vi "Test RT-TDMS-Logging API.vi"() -> ()   [LabVIEW 2021]
doc: "RT-TDMS-Logging API Tester."
uses:
  <vilib>/Utility/error.llb/DialogType.ctl
  RT-TDMS-Logging.lvlib
panel:
  in  "DO Data 2":variant
  in  "DO Data":bool
  in  "Start Logging 2":variant
  in  "Start Logging":bool
  in  "AI Data's 2":variant
  in  "AI Data's":bool
  in  "Data Logging Duration(Sec)":dbl
  in  "Data Logging Duration":bool
  out "last error":errorcluster
  in  "Show Diagram on Init":bool
  in  "Show Block Diagram":bool
  in  "Stop Module":bool
  in  "Start Module":bool
  in  "Hide Module Panel":bool
  in  "Show Module Panel":bool
  out "Status":string
  out "Module Running?":bool
  # "This VI tests the API for the Module."
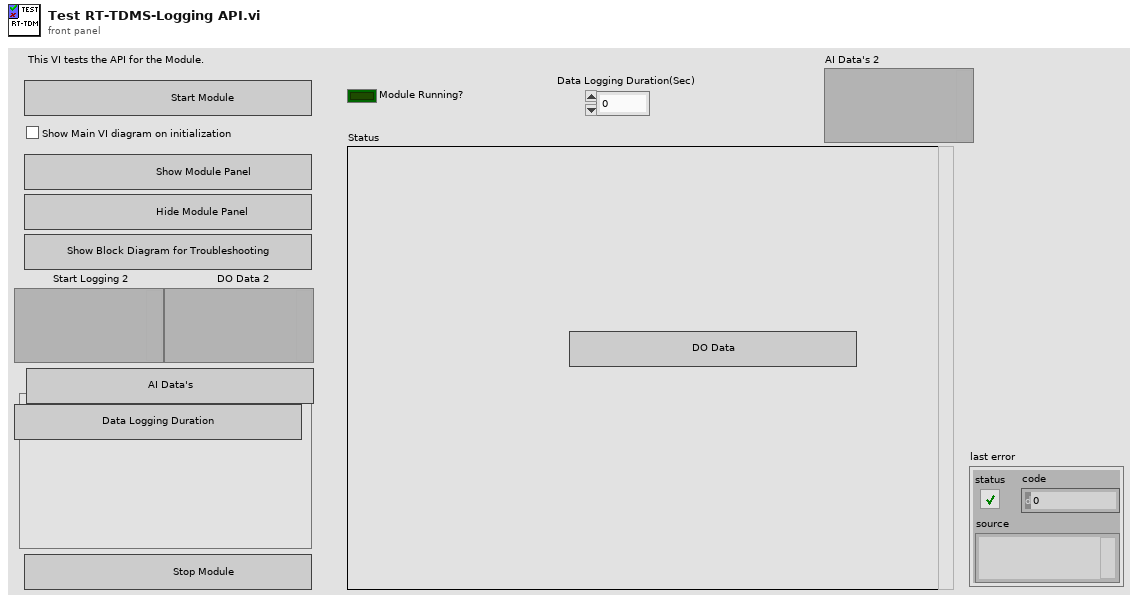
[diagram p1: front panel]
types:
  T1 = typedef "RT-TDMS-Logging.lvlib/Broadcast Events--cluster.ctl" = cluster{"Module Did Init":refnum<user-event>, "Status Updated":refnum<user-event>, "Error Reported":refnum<user-event>, "Module Did Stop":refnum<user-event>, "Update Module Execution Status":refnum<user-event>}
  T2 = typedef "DialogType.ctl" = u16
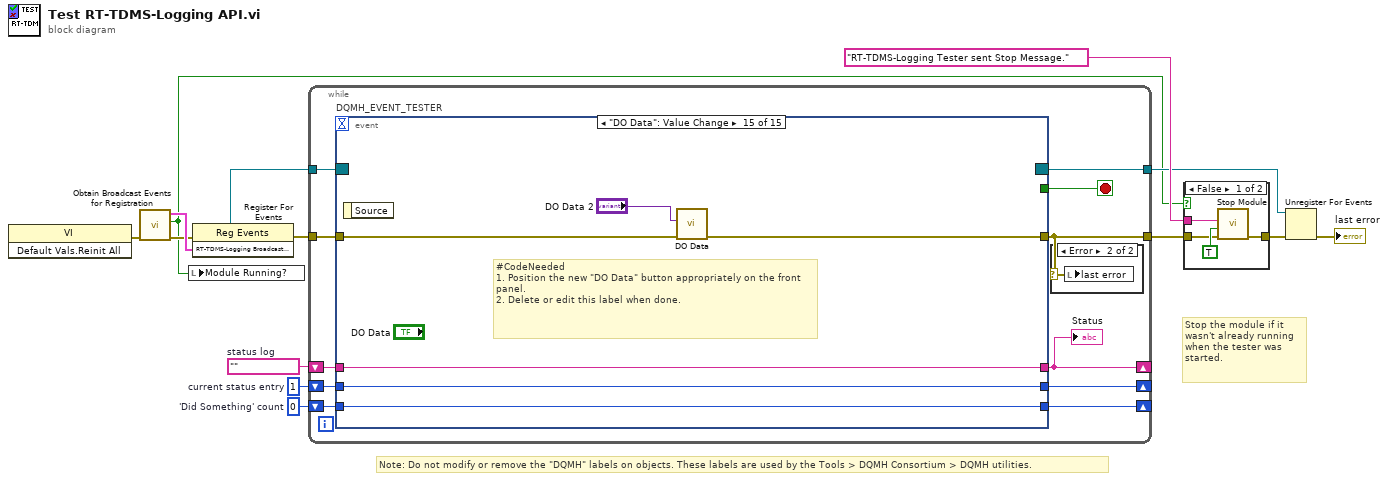
[diagram p0: block diagram]
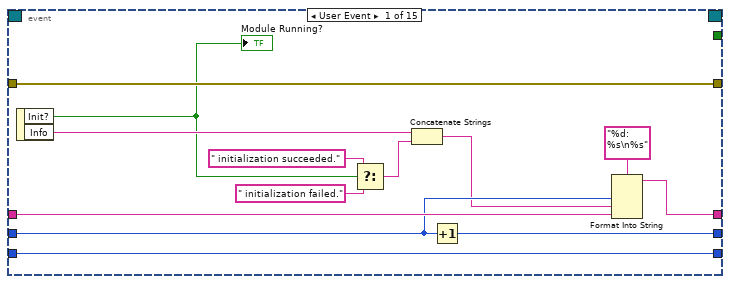
[diagram p4: hidden frame]
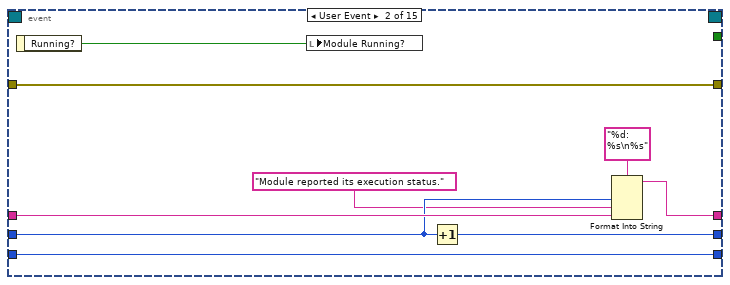
[diagram p5: hidden frame]
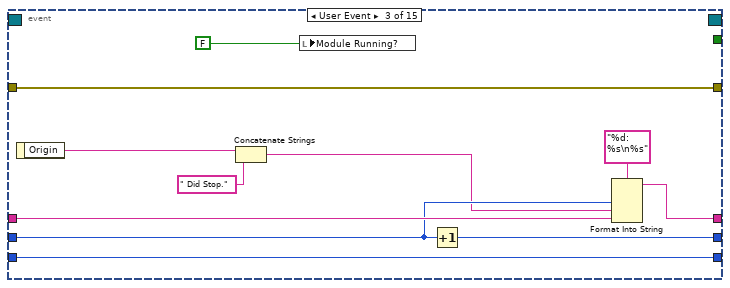
[diagram p6: hidden frame]
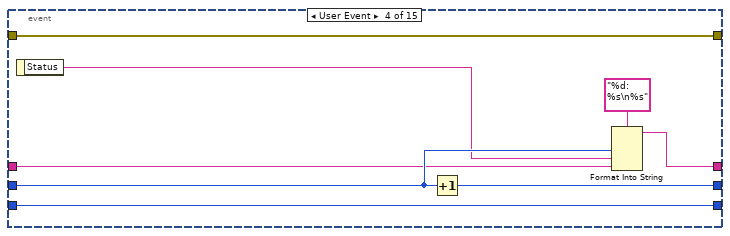
[diagram p7: hidden frame]
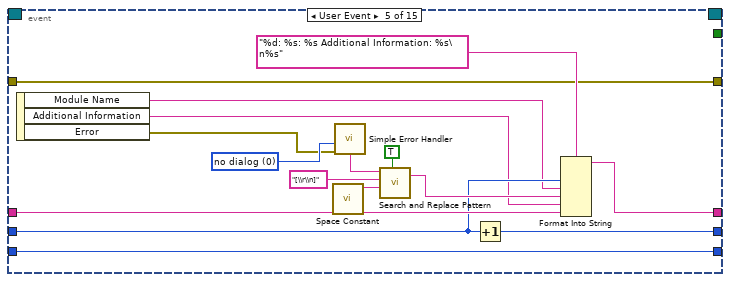
[diagram p8: hidden frame]
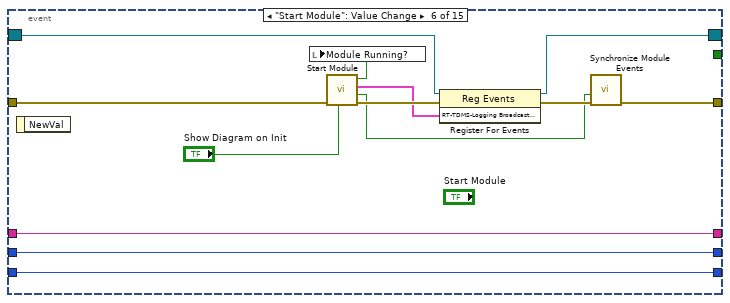
[diagram p9: hidden frame]
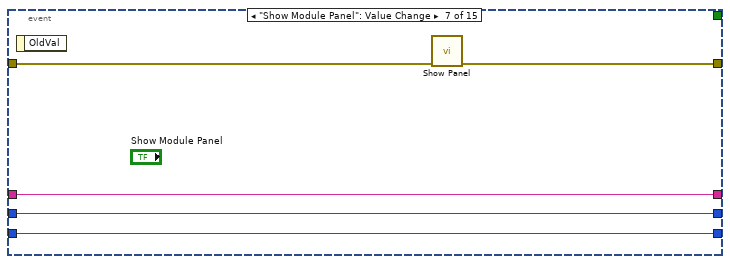
[diagram p10: hidden frame]
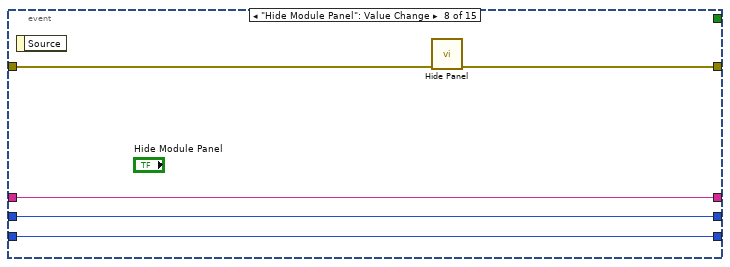
[diagram p11: hidden frame]
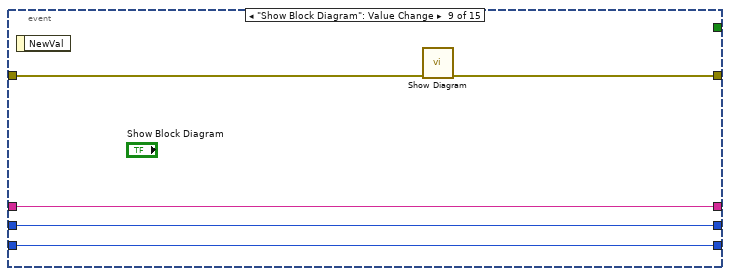
[diagram p12: hidden frame]
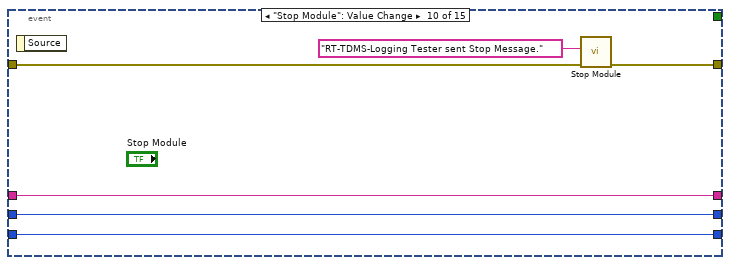
[diagram p13: hidden frame]
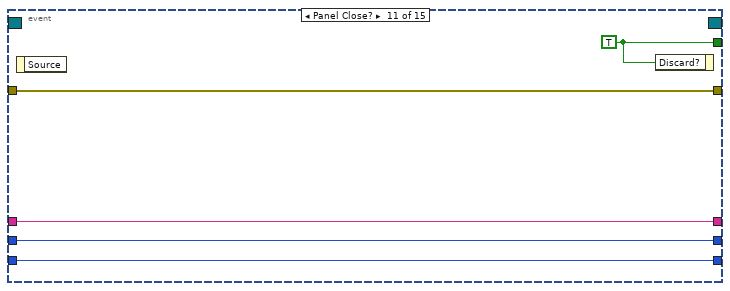
[diagram p14: hidden frame]
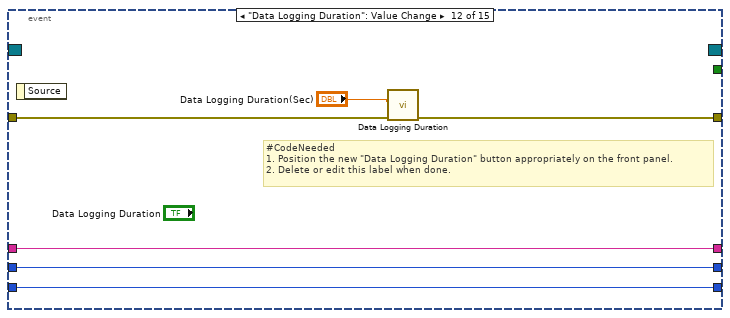
[diagram p15: hidden frame]
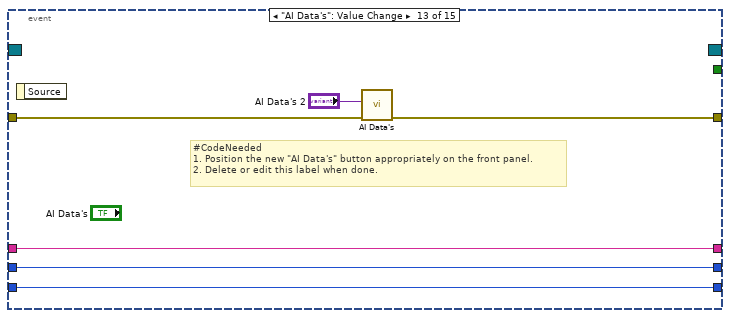
[diagram p16: hidden frame]
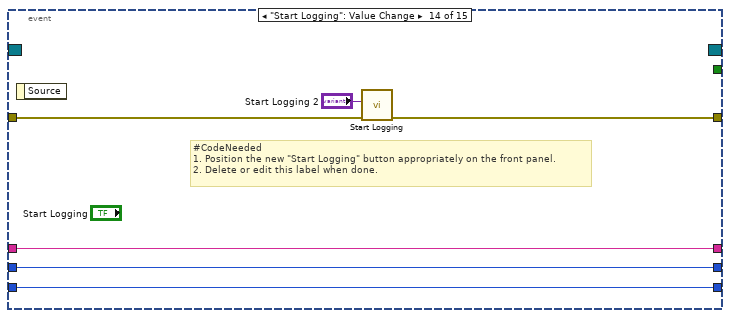
[diagram p17: hidden frame]
diagram:
  w10 = 0  # 'Did Something' count
  w11 = 1  # current status entry
  w12 = ""  # status log
  # "Stop the module if it wasn't already running when the tester was started."
  # "Note: Do not modify or remove the \"DQMH\" labels on objects. These labels are used by the Tools > DQMH Consortium > DQMH utilities."
  n1 = invoke class="VI" method="Default Vals.Reinit All"() -> (error out=w5:errorcluster)  [unwired: 3 in, 2 out]
  n2 = call "Obtain Broadcast Events for Registration.vi"("error in"=w5) -> ("error out"=w4:errorcluster, "Already running?"=w3:bool, "RT-TDMS-Logging Broadcast Events"=w8:T1)  [unwired: 8 in]
  n3 = local write "Module Running?"(w3) -> ()
  n4 = register-events(error in=w4, w8) -> (reference out=w7:refnum<event-registration>, error out=w9:errorcluster)  [unwired: 1 in]
  n5 = while {
    tunnel: w7 -> [w25]
    tunnel: [w15] -> w2
    shift-right: [w21] -> _
    shift-left: w12 -> [w23]
    shift-right: [w22] -> _
    shift-left: w11 -> [w24]
    shift-right: [w19] -> _
    shift-left: w10 -> [w20]
    tunnel: w9 -> [w18]
    tunnel: [w17] -> w6
    stop <- w16 stop-if-true
    n6 = event "DQMH_EVENT_TESTER" shown="[14] \"DO Data\": Value Change" {
      selector: w25 -> [_ _ _ _ _ w89 _ _ _ _ _ _ _ _ _]
      dyn-events: [_ _ _ _ _ w88 _ _ _ _ _ _ _ _ _] -> w17
      timeout: _ -> [_ _ _ _ _ _ _ _ _ _ _ _ _ _ _]
      tunnel: [_ _ _ _ _ _ _ _ _ _ w122 _ _ _ _] -> w16
      tunnel: [w39 w41 w49 w60 w71 w87 w101 w106 w107 w114 w118 w124 w130 w136 w142] -> w15
      tunnel: w24 -> [w36 w46 w57 w64 w74 w93 w99 w104 w109 w116 w120 w126 w132 w138 w144]
      tunnel: w23 -> [w37 w47 w58 w63 w75 w94 w100 w105 w110 w117 w121 w127 w133 w139 w145]
      tunnel: [w34 w44 w55 w65 w73 w94 w100 w105 w110 w117 w121 w127 w133 w139 w145] -> w21
      tunnel: [w35 w45 w56 w67 w72 w93 w99 w104 w109 w116 w120 w126 w132 w138 w144] -> w22
      tunnel: w20 -> [w31 w42 w51 w61 w83 w92 w98 w103 w108 w115 w119 w125 w131 w137 w143]
      tunnel: [w31 w42 w51 w61 w83 w92 w98 w103 w108 w115 w119 w125 w131 w137 w143] -> w19
      tunnel: w18 -> [w39 w41 w49 w60 w71 w86 w97 w102 w111 w112 w118 w128 w134 w140 w146]
      event User Event {
        n7 = event-data() -> ("Init?"=w30:bool, "Info"=w33:string)  [unwired: 1 in]
        "Module Running?" <- w30
        n8 = Select(t=" initialization succeeded.", s=w30, f=" initialization failed.") -> (s? t:f=w27:string)
        n9 = Concatenate Strings(w33, w27) -> (w32:string)
        n10 = Increment(x=w36) -> (x+1=w35:i32)
        n11 = Format Into String(format string="%d: %s\n%s", w36, w32, w37) -> (resulting string=w34:string)  [unwired: 2 in, 1 out]
      }
      event User Event {
        n12 = event-data() -> ("Running?"=w40:bool)  [unwired: 1 in]
        n13 = local write "Module Running?"(w40) -> ()
        n14 = Increment(x=w46) -> (x+1=w45:i32)
        n15 = Format Into String(format string="%d: %s\n%s", w46, "Module reported its execution status.", w47) -> (resulting string=w44:string)  [unwired: 2 in, 1 out]
      }
      event User Event {
        n16 = event-data() -> ("Origin"=w54:string)  [unwired: 1 in]
        n17 = Concatenate Strings(w54, " Did Stop.") -> (w53:string)
        n18 = local write "Module Running?"(FALSE ("Module Did Init?")) -> ()
        n19 = Increment(x=w57) -> (x+1=w56:i32)
        n20 = Format Into String(format string="%d: %s\n%s", w57, w53, w58) -> (resulting string=w55:string)  [unwired: 2 in, 1 out]
      }
      event User Event {
        n21 = event-data() -> ("Status"=w62:string)  [unwired: 1 in]
        n22 = Increment(x=w64) -> (x+1=w67:i32)
        n23 = Format Into String(format string="%d: %s\n%s", w64, w62, w63) -> (resulting string=w65:string)  [unwired: 2 in, 1 out]
      }
      event User Event {
        w76 = T2 0 items=["no dialog", "OK message", "continue or stop message", "OK message + warnings", "continue/stop + warnings"] ("type of dialog (OK msg:1)")
        n24 = event-data() -> ("Module Name"=w70:string, "Additional Information"=w69:string, "Error"=w68:errorcluster)  [unwired: 1 in]
        n25 = call <vilib>:"Space Constant.vi"() -> ("String"=w80:string)
        n26 = call <vilib>:"Simple Error Handler.vi"("type of dialog (OK msg:1)"=w76, "error in (no error)"=w68) -> ("message"=w77:string)  [unwired: 3 in, 4 out]
        n27 = call <vilib>:"Search and Replace Pattern.vi"("string"=w77, "regular expression (\"\")"="[\\r\\n]" ("regular expression (\"\")"), "replace string (\"\")"=w80, "replace all? (F)"=TRUE ("replace all CR/LF with spaces")) -> ("result string"=w78:string)  [unwired: 1 in, 1 out]
        n28 = Increment(x=w74) -> (x+1=w72:i32)
        n29 = Format Into String(format string="%d: %s: %s Additional Information: %s\n%s", w74, w70, w78, w69, w75) -> (resulting string=w73:string)  [unwired: 2 in, 1 out]
      }
      event "Start Module": Value Change {
        n30 = event-data() -> ()  [unwired: 1 in, 1 out]
        n31 = call "Start Module.vi"("Show Main VI Diagram on Init (F)"="Show Diagram on Init", "error in"=w86) -> ("error out"=w95:errorcluster, "Wait for Event Sync?"=w91:bool, "RT-TDMS-Logging Broadcast Events"=w90:T1, "Module Was Already Running?"=w85:bool)  [unwired: 6 in]
        n32 = local write "Module Running?"(w85) -> ()
        n33 = register-events(reference=w89, error in=w95, w90) -> (reference out=w88:refnum<event-registration>, error out=w96:errorcluster)
        n34 = call "Synchronize Module Events.vi"("error in"=w96, "Wait for Event Sync?"=w91) -> ("error out"=w87:errorcluster)  [unwired: 9 in]
      }
      event "Show Module Panel": Value Change {
        n35 = event-data() -> ()  [unwired: 1 in, 1 out]
        n36 = call "Show Panel.vi"("error in"=w97) -> ("error out"=w101:errorcluster)  [unwired: 10 in]
      }
      event "Hide Module Panel": Value Change {
        n37 = event-data() -> ()  [unwired: 1 in, 1 out]
        n38 = call "Hide Panel.vi"("error in"=w102) -> ("error out"=w106:errorcluster)  [unwired: 10 in]
      }
      event "Show Block Diagram": Value Change {
        n39 = event-data() -> ()  [unwired: 1 in, 1 out]
        n40 = call "Show Diagram.vi"("error in"=w111) -> ("error out"=w107:errorcluster)  [unwired: 10 in]
      }
      event "Stop Module": Value Change {
        n41 = event-data() -> ()  [unwired: 1 in, 1 out]
        n42 = call "Stop Module.vi"("error in"=w112, "Origin"="RT-TDMS-Logging Tester sent Stop Message.") -> ("error out"=w114:errorcluster)  [unwired: 9 in]
      }
      event Panel Close? {
        w122 = TRUE ("Discard?")
        n43 = event-data() -> ()  [unwired: 1 in, 1 out]
        n44 = event-data("Discard?"=w122) -> ()  [unwired: 1 in, 1 out]
      }
      event "Data Logging Duration": Value Change {
        # "#CodeNeeded\n1. Position the new \"Data Logging Duration\" button appropriately on the front panel.\n2. Delete or edit this label when done."
        n45 = event-data() -> ()  [unwired: 1 in, 1 out]
        n46 = call "Data Logging Duration.vi"("error in"=w128, "Data Logging Duration(Sec)"="Data Logging Duration(Sec)") -> ("error out"=w124:errorcluster)  [unwired: 9 in]
      }
      event "AI Data's": Value Change {
        # "#CodeNeeded\n1. Position the new \"AI Data's\" button appropriately on the front panel.\n2. Delete or edit this label when done."
        n47 = event-data() -> ()  [unwired: 1 in, 1 out]
        n48 = call "AI Data's.vi"("error in"=w134, "AI Data's"="AI Data's 2") -> ("error out"=w130:errorcluster)  [unwired: 9 in]
      }
      event "Start Logging": Value Change {
        # "#CodeNeeded\n1. Position the new \"Start Logging\" button appropriately on the front panel.\n2. Delete or edit this label when done."
        n49 = event-data() -> ()  [unwired: 1 in, 1 out]
        n50 = call "Start Logging.vi"("error in"=w140, "Start Logging"="Start Logging 2") -> ("error out"=w136:errorcluster)  [unwired: 9 in]
      }
      event "DO Data": Value Change {
        # "#CodeNeeded\n1. Position the new \"DO Data\" button appropriately on the front panel.\n2. Delete or edit this label when done."
        n51 = event-data() -> ()  [unwired: 1 in, 1 out]
        n52 = call "DO Data.vi"("error in"=w146, "DO Data"="DO Data 2") -> ("error out"=w142:errorcluster)  [unwired: 9 in]
      }
    }
    "Status" <- w21
    n53 = case shown="Error" w15 {
      selector: w15 -> [_ w26]
      frame No Error {
      }
      frame Error {
        n54 = local write "last error"(w26) -> ()
      }
    }
  }
  n55 = case shown="False" w3 {
    tunnel: [w150 w151] -> w14
    tunnel: "RT-TDMS-Logging Tester sent Stop Message." ("Origin") -> [w149 _]
    tunnel: w2 -> [w147 w151]
    frame False {
      n56 = call "Stop Module.vi"("error in"=w147, "Wait for Module to Stop? (F)"=TRUE ("Wait for Module to stop?"), "Origin"=w149) -> ("error out"=w150:errorcluster)  [unwired: 8 in]
    }
    frame True {
    }
  }
  n57 = Unregister For Events(event registration refnum=w6, error in=w14) -> (error out=→"last error":errorcluster)
